vi "CPUload.vi"() -> (2 "process time":dbl format="%<%H:%M:%S%3u>t", 4 "return":i32)   [LabVIEW 2016]
uses:
  processHandles.dll
panel:
  out "processor time":dbl
  out "Total user and kernel":dbl format="%<%H:%M:%S%3u>t"
  out "Idle time":dbl format="%<%H:%M:%S%3u>t"
  out "total user":T1
  out "total kernel":T1
  out "Idle":T1
  in  "Cluster 7":T1
  in  "Cluster 6":T1
  in  "Cluster 5":T1
  out "lpUserTime":T1
  out "lpKernelTime":T1
  out "lpExitTime":T1
  out "lpCreationTime":T1
  in  "Cluster 4":T1
  in  "Cluster 3":T1
  in  "Cluster 2":T1
  in  "Cluster":T1
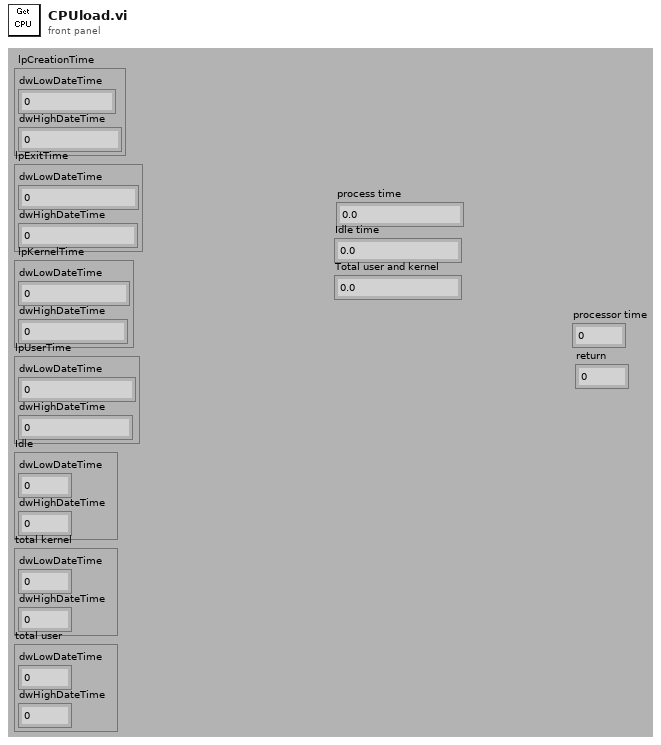
[diagram p1: front panel]
types:
  T1 = cluster{"dwLowDateTime":u32, "dwHighDateTime":u32}
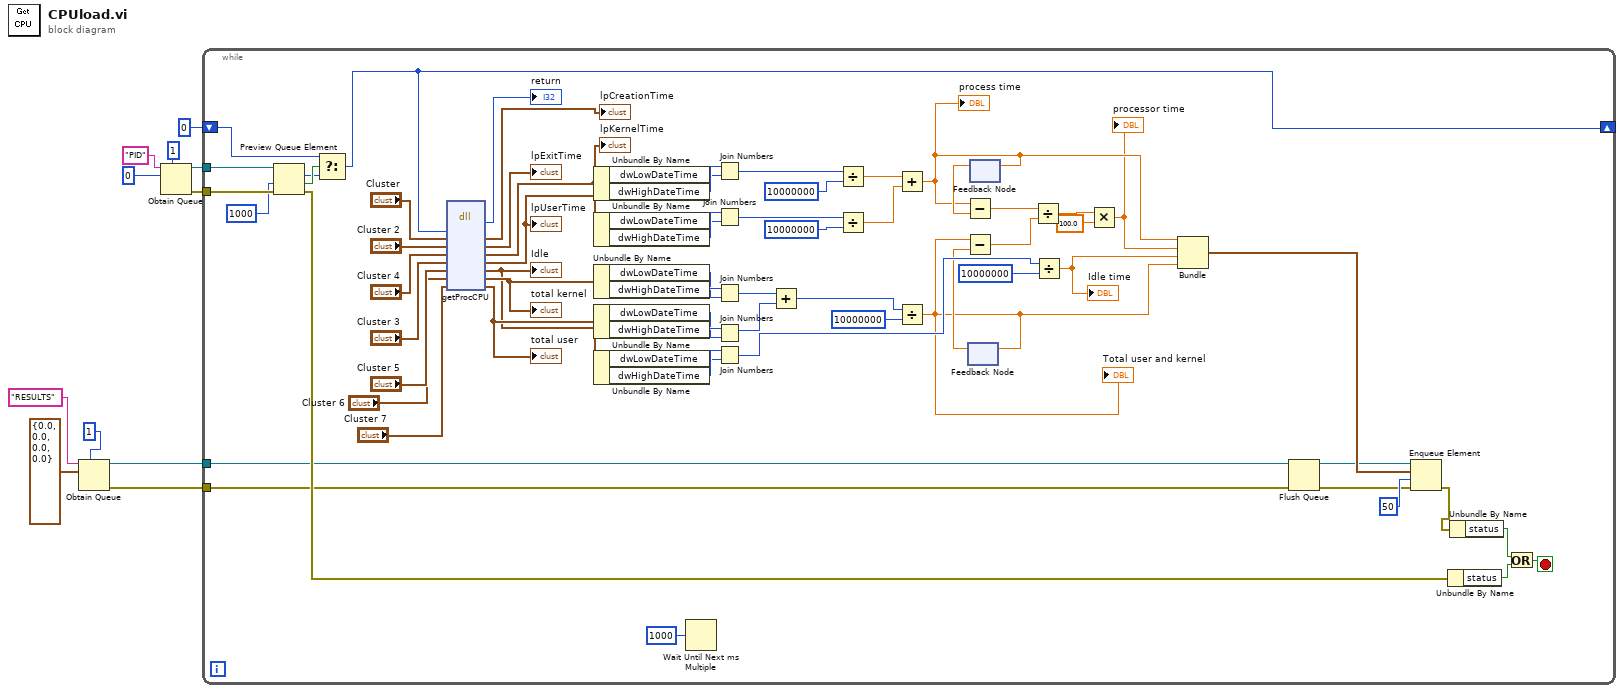
[diagram p0: block diagram]
diagram:
  n1 = Obtain Queue(max queue size (-1, unlimited)=1, name (unnamed)="RESULTS", element data type=cluster{dbl, dbl, dbl, dbl} {0.0, 0.0, 0.0, 0.0}) -> (queue out=w4:refnum<queue>, error out=w3:errorcluster)  [unwired: 2 in, 1 out]
  n2 = Obtain Queue(max queue size (-1, unlimited)=1, name (unnamed)="PID", element data type=0) -> (queue out=w11:refnum<queue>, error out=w10:errorcluster)  [unwired: 2 in, 1 out]
  n3 = while {
    tunnel: w11 -> [w34]
    tunnel: w10 -> [w33]
    shift-right: [w28] -> _
    shift-left: 0 -> [w30]
    tunnel: w4 -> [w16]
    tunnel: w3 -> [w15]
    stop <- w18 stop-if-true
    n4 = Preview Queue Element(queue=w34, timeout in ms (-1)=u32 1000 ("millisecond multiple"), error in (no error)=w33) -> (element=w29:i32, timed out?=w31:bool, error out=w21:errorcluster)  [unwired: 1 out]
    n5 = Select(t=w30, s=w31, f=w29) -> (s? t:f=w28:i32)
    n6 = dll-call lib="C:/Technology Lab/NI-2010/Trunk/Utility/Project Memory Manager/Project Manager/processHandles.dll" fn="getProcCPU"("arg5"=w28, "arg1"="Cluster", "arg2"="Cluster 2", "arg3"="Cluster 4", "arg4"="Cluster 3", "arg6"="Cluster 5", "arg7"="Cluster 6", "arg8"="Cluster 7") -> ("return type"=→"return":i32, "arg1"=→"lpCreationTime":T1, "arg2"=→"lpExitTime":T1, "arg3"=w70:T1, "arg4"=w67:T1, "arg6"=w49:T1, "arg7"=w53:T1, "arg8"=w52:T1)  [unwired: 4 in, 2 out]
    "lpKernelTime" <- w70
    "lpUserTime" <- w67
    "Idle" <- w49
    "total kernel" <- w53
    "total user" <- w52
    n7 = Unbundle By Name(w70) -> ("dwLowDateTime"=w68:u32, "dwHighDateTime"=w69:u32)
    n8 = Unbundle By Name(w67) -> ("dwLowDateTime"=w65:u32, "dwHighDateTime"=w66:u32)
    n9 = Unbundle By Name(w53) -> ("dwLowDateTime"=w55:u32, "dwHighDateTime"=w57:u32)
    n10 = Unbundle By Name(w52) -> ("dwLowDateTime"=w54:u32, "dwHighDateTime"=w56:u32)
    n11 = Unbundle By Name(w49) -> ("dwLowDateTime"=w47:u32, "dwHighDateTime"=w48:u32)
    n12 = Wait Until Next ms Multiple(millisecond multiple=u32 1000) -> ()  [unwired: 1 out]
    n13 = Join Numbers(hi=w69, lo=w68) -> ((hi.lo)=w46:u64)
    n14 = Join Numbers(hi=w66, lo=w65) -> ((hi.lo)=w45:u64)
    n15 = Join Numbers(hi=w57, lo=w55) -> ((hi.lo)=w50:u64)
    n16 = Join Numbers(hi=w56, lo=w54) -> ((hi.lo)=w51:u64)
    n17 = Join Numbers(hi=w48, lo=w47) -> ((hi.lo)=w44:u64)
    n18 = Add(x=w50, y=w51) -> (x+y=w42:u64)
    n19 = Divide(x=w46, y=u64 10000000) -> (x/y=w62:dbl)
    n20 = Divide(x=w45, y=u64 10000000) -> (x/y=w61:dbl)
    n21 = Add(x=w62, y=w61) -> (x+y=w27:dbl)
    "process time" <- w27
    n22 = Divide(x=w42, y=u64 10000000) -> (x/y=w24:dbl)
    "Total user and kernel" <- w24
    n23 = feedback-in #1(w24) -> ()
    n24 = feedback #1() -> (w35:dbl)  [unwired: 1 in]
    n25 = Subtract(x=w24, y=w35) -> (x-y=w36:dbl)
    n26 = feedback-in #2(w27) -> ()
    n27 = feedback #2() -> (w40:dbl)  [unwired: 1 in]
    n28 = Subtract(x=w27, y=w40) -> (x-y=w39:dbl)
    n29 = Divide(x=w39, y=w36) -> (x/y=w38:dbl)
    n30 = Divide(x=w44, y=u64 10000000) -> (x/y=w25:dbl)
    "Idle time" <- w25
    n31 = Multiply(x=w38, y=100.0) -> (x*y=w26:dbl)
    "processor time" <- w26
    n32 = Bundle(w27, w26, w25, w24) -> (w23:cluster{dbl, dbl, dbl, dbl})  [unwired: 1 in]
    n33 = Flush Queue(queue=w16, error in (no error)=w15) -> (queue out=w13:refnum<queue>, error out=w14:errorcluster)  [unwired: 1 out]
    n34 = Enqueue Element(queue=w13, element=w23, timeout in ms (-1)=50, error in (no error)=w14) -> (error out=w22:errorcluster)  [unwired: 2 out]
    n35 = Unbundle By Name(w21) -> ("status"=w20:bool)
    n36 = Unbundle By Name(w22) -> ("status"=w19:bool)
    n37 = Or(x=w19, y=w20) -> (x .or. y?=w18:bool)
  }
